vi "Init Stream.vi"(8 "error in (no error)":errorcluster, 11 "Channel in":refnum<class "Channel.lvclass">) -> (0 "error out":errorcluster, 3 "Channel out":refnum<class "Channel.lvclass">)   [LabVIEW 2018, in "Channel.lvclass"]
uses:
  Channel.lvclass
  Channel.lvclass/Channel.ctl
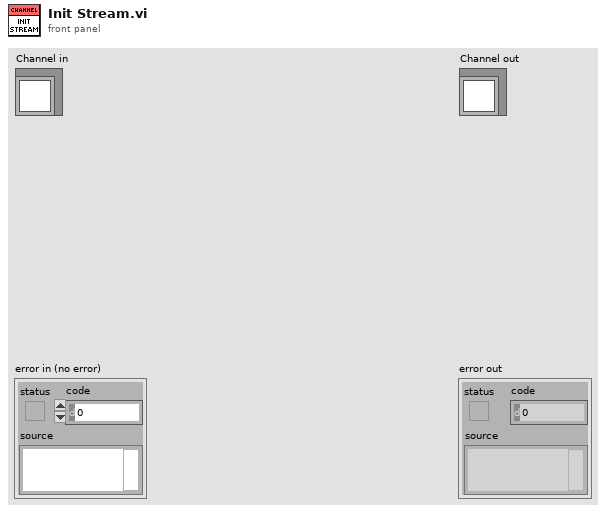
[diagram p1: front panel]
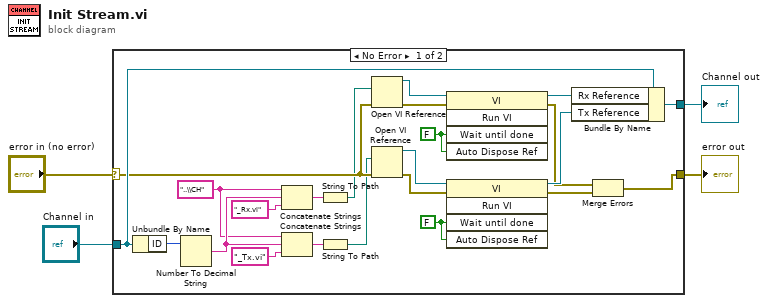
[diagram p0: block diagram]
diagram:
  n1 = case shown="No Error" "error in (no error)" {
    selector: "error in (no error)" -> [w11 w29]
    tunnel: [w14 w29] -> w2
    tunnel: [w23 w28] -> w1
    tunnel: "Channel in" -> [w24 w28]
    frame No Error {
      w20 = FALSE ("Wait Until Done")
      w9 = "..\\CH" ("name or relative path")
      w26 = FALSE ("Wait Until Done")
      n2 = Unbundle By Name(w24) -> ("ID"=w10:u16)
      n3 = Number To Decimal String(number=w10) -> (decimal integer string=w18:string)  [unwired: 1 in]
      n4 = Concatenate Strings(w9, w18, "_Rx.vi" ("name or relative path")) -> (w7:string)
      n5 = Concatenate Strings(w9, w18, "_Tx.vi" ("name or relative path")) -> (w6:string)
      n6 = String To Path(string=w7) -> (path=w8:path)
      n7 = String To Path(string=w6) -> (path=w5:path)
      n8 = Open VI Reference(vi path=w8, error in (no error)=w11) -> (vi reference=w27:refnum<vi>, error out=w13:errorcluster)  [unwired: 4 in]
      n9 = Open VI Reference(vi path=w5, error in (no error)=w11) -> (vi reference=w19:refnum<vi>, error out=w12:errorcluster)  [unwired: 4 in]
      n10 = invoke class="VI" method="Run VI"(reference=w27, error in=w13, "Wait until done"=w26, "Auto Dispose Ref"=w26) -> (reference out=w22:refnum<vi>, error out=w15:errorcluster)  [unwired: 1 in, 3 out]
      n11 = invoke class="VI" method="Run VI"(reference=w19, error in=w12, "Wait until done"=w20, "Auto Dispose Ref"=w20) -> (reference out=w17:refnum<vi>, error out=w16:errorcluster)  [unwired: 1 in, 3 out]
      n12 = Bundle By Name(cluster=w24, "Rx Reference"=w22, "Tx Reference"=w17) -> (w23:refnum<class "Channel.lvclass">)
      n13 = Merge Errors(w15, w16) -> (w14:errorcluster)
    }
    frame Error {
    }
  }
  "error out" <- w2
  "Channel out" <- w1
